vi "encoding_(subvi).vi"(6 "y1 in":dbl, 7 "beam waist w0 (m) in":dbl=0.0001 format="%.2p", 9 "y0 in":dbl, 10 "d in":dbl, 11 "beam parameters in":T1) -> (3 "mode superposition 2":T1)   [LabVIEW 2015]
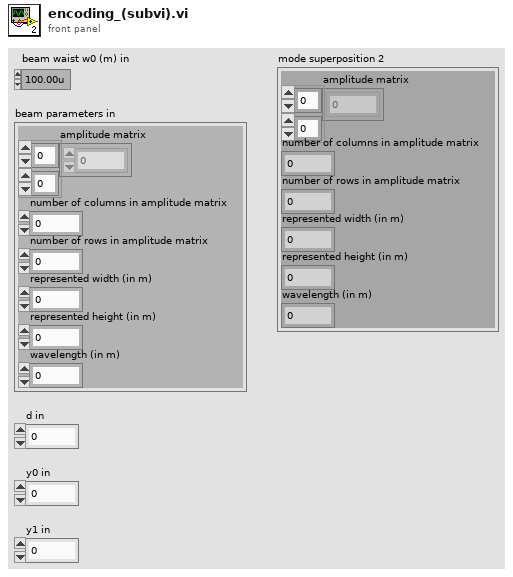
[diagram p1: front panel]
types:
  T1 = cluster{"amplitude matrix":cdb[][], "number of columns in amplitude matrix":i32, "number of rows in amplitude matrix":i32, "represented width (in m)":dbl, "represented height (in m)":dbl, "wavelength (in m)":dbl}
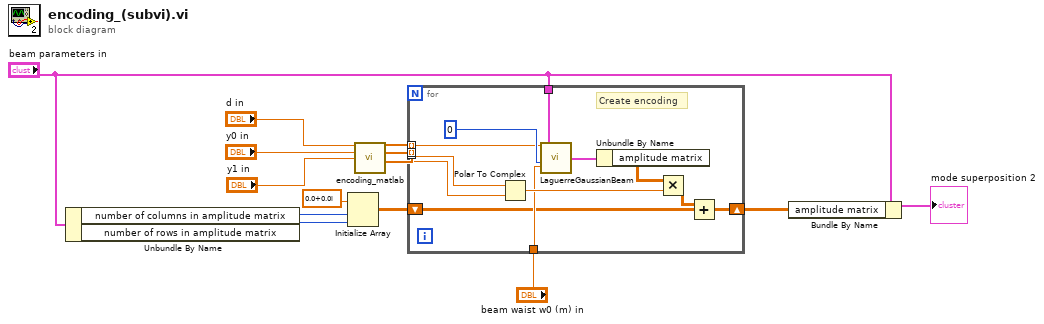
[diagram p0: block diagram]
diagram:
  n1 = Unbundle By Name("beam parameters in") -> ("number of columns in amplitude matrix"=w11:i32, "number of rows in amplitude matrix"=w12:i32)
  n2 = Initialize Array(cdb 0.0+0.0i ("element"), w11, w12) -> (w3:cdb[][])
  n3 = call "encoding_matlab.vi"("d"="d in", "y0"="y0 in", "y1"="y1 in") -> ("modes"=w5:dbl[], "coeffs"=w6:dbl[], "phase"=w7:dbl[])  [unwired: 10 in]
  n4 = for {
    tunnel: "beam parameters in" -> [w23]
    tunnel: "beam waist w0 (m) in" -> [w22]
    shift-right: [w19] -> w4
    shift-left: w3 -> [w20]
    tunnel: w5 -> [w17] mode=indexing
    tunnel: w6 -> [w15] mode=indexing
    tunnel: w7 -> [w16] mode=indexing
    # "Create encoding"
    n5 = Polar To Complex(1:w16, 2:w15) -> (0:w24:cdb)
    n6 = call <userlib>:"LaguerreGaussianBeam.vi"("beam waist w0 (in m; default 1E-4 = 0.1mm)"=w22, "p"=0, "l"=w17, "beam parameters"=w23) -> ("Laguerre-Gaussian beam"=w18:T1)  [unwired: 7 in]
    n7 = Unbundle By Name(w18) -> ("amplitude matrix"=w25:cdb[][])
    n8 = Multiply(x=w25, y=w24) -> (x*y=w21:cdb[][])
    n9 = Add(x=w21, y=w20) -> (x+y=w19:cdb[][])
  }
  n10 = Bundle By Name(cluster="beam parameters in", "amplitude matrix"=w4) -> (→"mode superposition 2":T1)
